vi "Update Trace.vi"(8 "Error In":errorcluster, 11 "Pixel In":refnum<class "Pixel.lvclass">) -> (0 "Error Out":errorcluster, 3 "Pixel Out":refnum<class "Pixel.lvclass">)   [LabVIEW 2019, in "Pixel.lvclass"]
uses:
  Pixel.lvclass
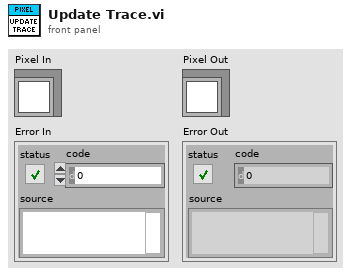
[diagram p1: front panel]
types:
  T1 = typedef "Display Element.lvclass/Vector.ctl" = cluster{"X":i32, "Y":i32}
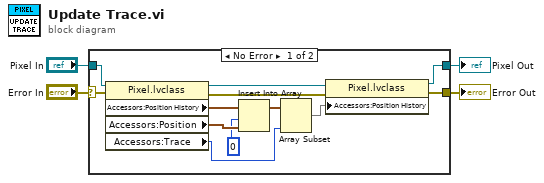
[diagram p0: block diagram]
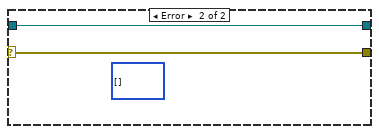
[diagram p2: hidden frame]
diagram:
  n1 = case shown="No Error" "Error In" {
    selector: "Error In" -> [w13 w18]
    tunnel: "Pixel In" -> [w14 w17]
    tunnel: [w16 w18] -> w2
    tunnel: [w15 w17] -> w1
    frame No Error {
      n2 = property class="Pixel.lvclass"(reference=w14, error in=w13) -> (reference out=w12:refnum<class "Pixel.lvclass">, error out=w11:errorcluster, "Accessors:Position History"=w10:T1[], "Accessors:Position"=w9:T1, "Accessors:Trace"=w6:i32)
      n3 = Insert Into Array(array=w10, index=0, new element=w9) -> (w7:T1[])
      n4 = Array Subset(array=w7, length=w6) -> (w5:T1[])  [unwired: 1 in]
      n5 = property class="Pixel.lvclass"(reference=w12, error in=w11, "Accessors:Position History"=w5) -> (reference out=w15:refnum<class "Pixel.lvclass">, error out=w16:errorcluster)
    }
    frame Error {
      (unwired) u32[][] []
    }
  }
  "Pixel Out" <- w1
  "Error Out" <- w2
